vi "Level (G3) - Defaults.vi"() -> (1 "units mask":bool[](array[boolean]), 2 "valid units":T1[](array[typedef]), 3 "unit strings":string[](array[string]))   [LabVIEW 2020, in "Level (G3).xctl"]
uses:
  Level (G3).xctl
  Level Units (G3).ctl
panel:
  in  "Units":T1
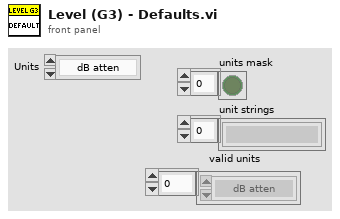
[diagram p1: front panel]
types:
  T1 = typedef "Level (G3).xctl/Level Units (G3).ctl" = enum16{"dB atten", "dB SPL", "dB re 1 Vrms", "dB V/Hz½", "mW", "dB HL", "Volts", "dB mW"}
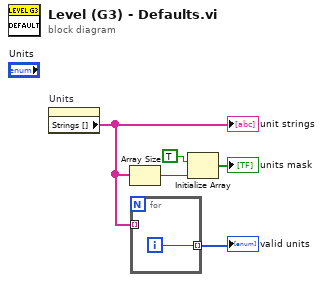
[diagram p0: block diagram]
diagram:
  n1 = property on="Units" class="Enum (strict)"() -> ("Strings []"=w2:string[])  [unwired: 2 in, 2 out]
  "unit strings" <- w2
  n2 = Array Size(array=w2) -> (size(s)=w5:i32)
  n3 = for {
    tunnel: w2 -> [_] mode=indexing
    tunnel: [w6] -> w1 mode=indexing
    i -> [w6]
  }
  "valid units" <- w1
  n4 = Initialize Array(TRUE, w5) -> (→"units mask":bool[])
